vi "_Test_MMAPI_Receive.vi"() -> ()   [LabVIEW 2023]
uses:
  Shared/SensorInfos.ctl
  Shared/SensorInfo.ctl
  Shared/Sensor Name.ctl
  Shared/Protocol.ctl
  MM/MM Data.ctl
  MM/MM Objects.ctl
  MM/MM Object.ctl
  <vilib>/Utility/xml.llb/Read From XML File(string).vi
  <vilib>/xnet/xnet.llb/XNET Convert (Frame FlexRay to Signal).vi
  RDB/RDB.lvlib
  Shared/Vires VTD Shared.lvlib
  MM/MM.lvlib
  Utility/Debug_Logger/LoggingProber.lvlib
panel:
  in  "mmanager":path=path "C:/dev/Hexagon-VTD-Custom-Device/Libraries/libMM.dll"
  out "sensorInfos":T1
  out "size(s) 2":i32
  out "Array 2":u8[](array[numeric])
  out "Array":i32[](array[numeric])
  out "signal data":dbl[](array[numeric])
  out "simTime":dbl
  out "simFrame":dbl
  in  "XML File Path":path=path "C:/Debug/MM.xml"
  out "error out":errorcluster
  in  "error in (no error)":errorcluster
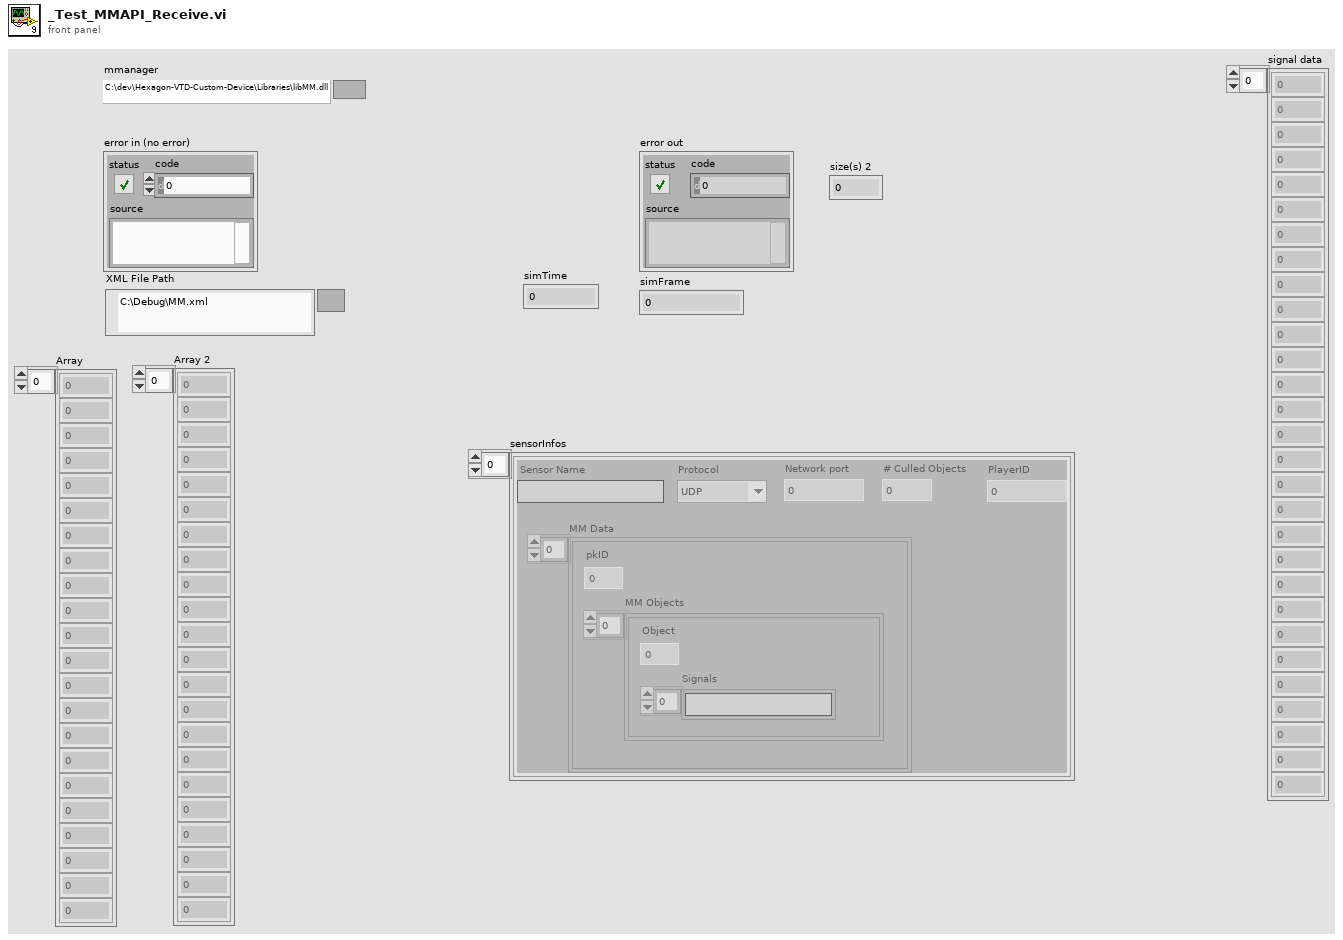
[diagram p1: front panel]
types:
  T1 = typedef "Vires VTD Shared.lvlib/SensorInfos.ctl" = T2[]
  T2 = typedef "Vires VTD Shared.lvlib/SensorInfo.ctl" = cluster{"Sensor Name":T3, "Protocol":T4, "Network port":i32, "# Culled Objects":i32, "PlayerID":u8, "MM Data":T5}
  T3 = typedef "Vires VTD Shared.lvlib/Sensor Name.ctl" = string
  T4 = typedef "Vires VTD Shared.lvlib/Protocol.ctl" = enum16{"UDP", "TCP"}
  T5 = typedef "Vires VTD Shared.lvlib/MM Data.ctl" = T6[]
  T6 = typedef "MM.lvlib/MM Objects.ctl" = cluster{"pkID":i32, "MM Objects":T7[]}
  T7 = typedef "MM.lvlib/MM Object.ctl" = cluster{"Object":i32, "Signals":string[]}
  T8 = typedef "MM.lvlib/Sensor Engine Data.ctl" = cluster{"TCP Network":refnum<k5>, "UDP Network":refnum<k16>, "Network port":i32, "Protocol":T4, "Sensor Name":T3, "Signal Data":dbl[], "MM Frames":T9[], "MM Culled Objects":i32[], "MM Frame Refs":refnum<k21>[], "mmanager":path, "mmHandle":u64}
  T9 = typedef "XNET Frame FlexRay.ctl" = cluster{"timestamp":timestamp, "payload":u8[], "slot":u16, "type":T10, "cycle count":u8, "startup?":bool, "sync?":bool, "preamble?":bool, "ch A":bool, "ch B":bool, "echo?":bool}
  T10 = typedef "XNET Frame Type FlexRay.ctl" = u8
  T11 = enum16{"Standard", "Buffered", "CRLF", "Immediate"}
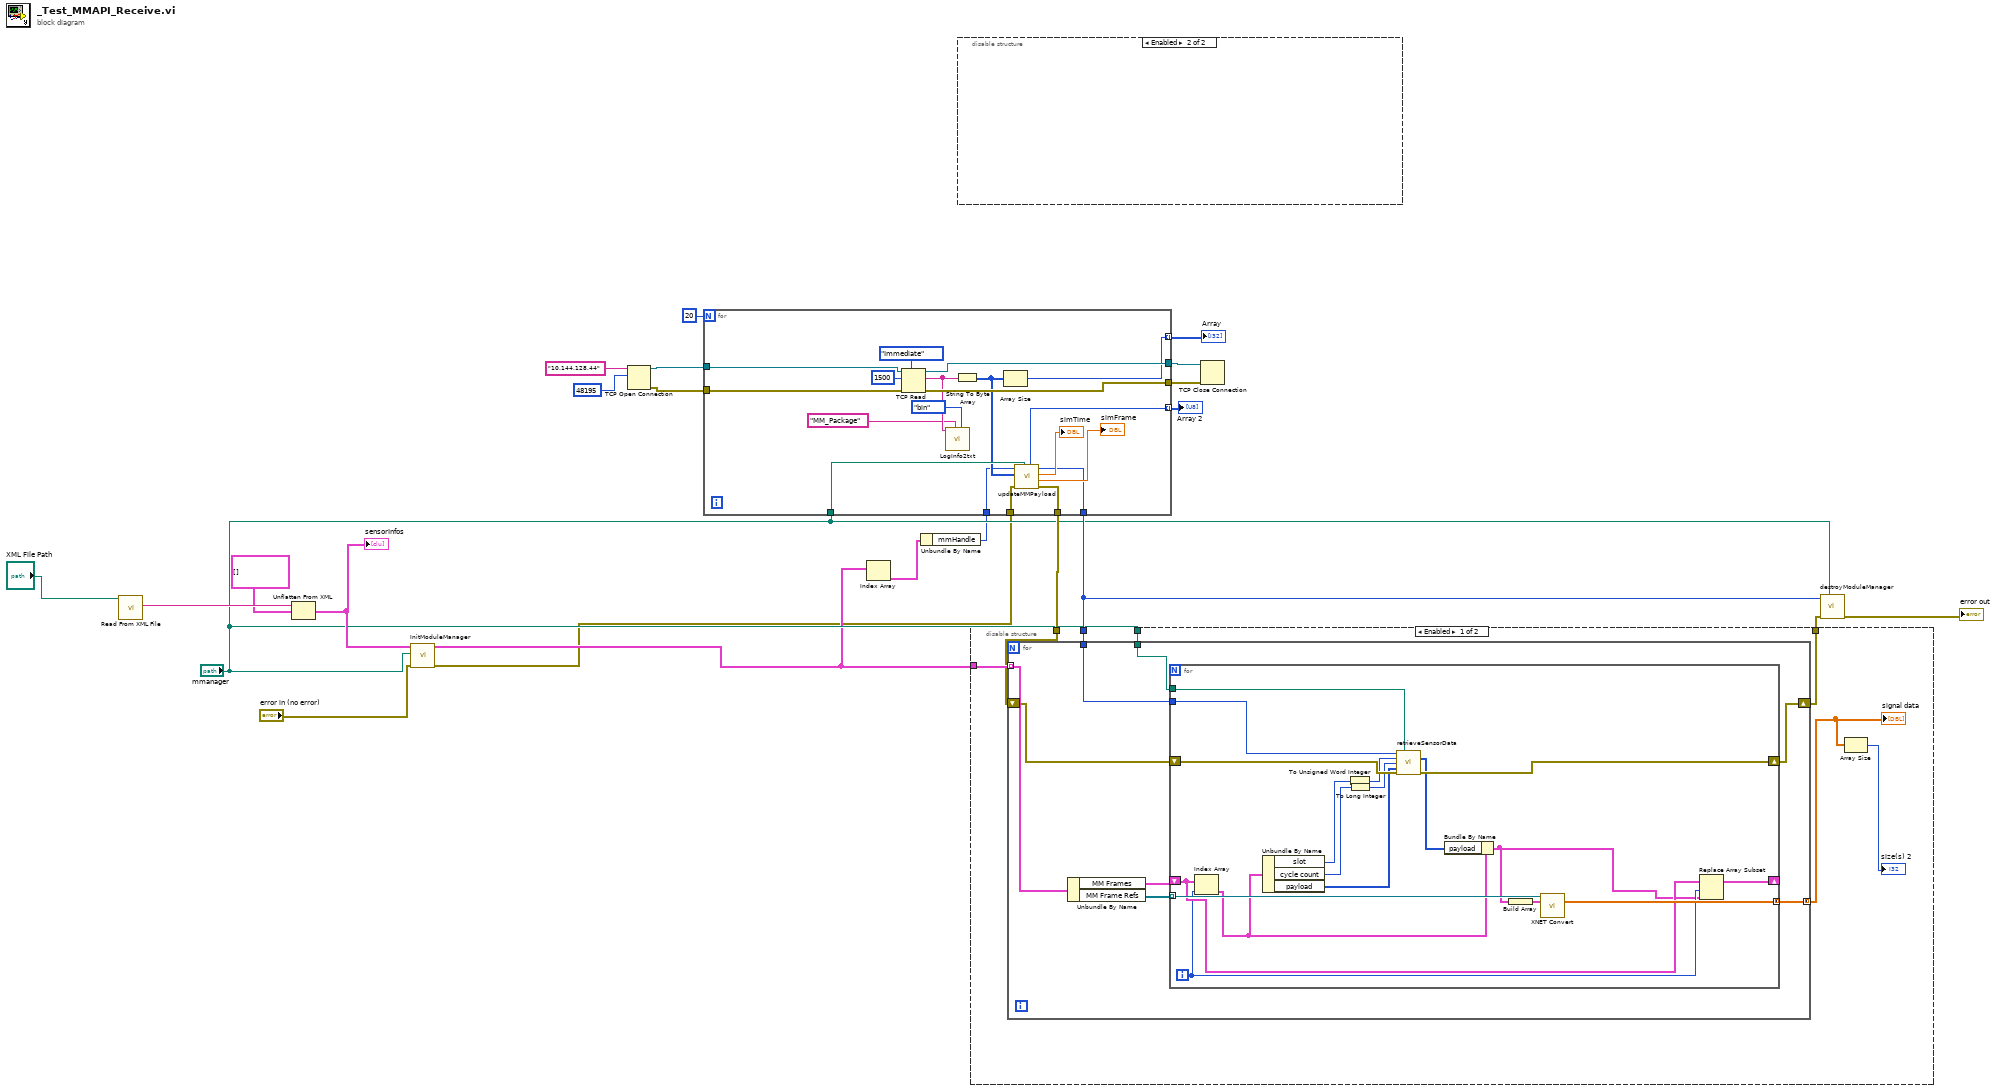
[diagram p0: block diagram]
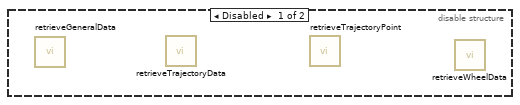
[diagram p3: hidden frame]
diagram:
  n1 = call-poly <vilib>:"Read From XML File.vi"("XML File Path"="XML File Path") -> ("XML Elements"=w23:string)  [unwired: 8 in, 2 out]
  n2 = Unflatten From XML(xml string=w23, type=T1 [] ("SensorInfos")) -> (value=w12:T1)  [unwired: 1 in, 1 out]
  "sensorInfos" <- w12
  n3 = call "InitModuleManager.vi"("error in (no error)"="error in (no error)", "mmanager"="mmanager", "SensorInfos"=w12) -> ("error out (no error)"=w1:errorcluster, "Sensor Engine Datas"=w5:T8[])  [unwired: 7 in]
  n4 = TCP Open Connection(address="10.144.128.44", remote port or service name=u16 48195) -> (connection ID=w18:refnum<k5>, error out=w19:errorcluster)  [unwired: 3 in]
  n5 = Index Array(array=w5) -> (element=w4:T8)  [unwired: 1 in]
  n6 = Unbundle By Name(w4) -> ("mmHandle"=w3:u64)
  n7 = for {
    N: 20 -> [_]
    tunnel: "mmanager" -> [w35]
    tunnel: w19 -> [w40]
    tunnel: w18 -> [w39]
    tunnel: [w38] -> w17
    tunnel: [w37] -> w16
    tunnel: [w36] -> w14 mode=indexing
    tunnel: w1 -> [w34]
    tunnel: [w32] -> w11 mode=indexing
    tunnel: [w29] -> w10
    tunnel: [w28] -> w7
    tunnel: w3 -> [w27]
    n8 = TCP Read(connection ID=w39, bytes to read=1500, error in (no error)=w40, 7:T11."Immediate" ("mode (standard)")) -> (connection ID out=w38:refnum<k5>, data out=w26:string, error out=w37:errorcluster)  [unwired: 1 in]
    n9 = call "LogInfo2txt.vi"("type"=enum16{"txt", "bin"}."bin", "File ID"="MM_Package", "text"=w26) -> ()  [unwired: 9 in]
    n10 = String To Byte Array(string=w26) -> (unsigned byte array=w33:u8[])
    n11 = Array Size(array=w33) -> (size(s)=w36:i32)
    n12 = call "updateMMPayload.vi"("path in"=w35, "error in (no error)"=w34, "payload"=w33, "mmHandle in"=w27) -> ("error out"=w29:errorcluster, "simFrame"=→"simFrame":dbl, "simTime"=→"simTime":dbl, "mmHandle out"=w28:u64, "isComplete"=w32:u8)  [unwired: 2 in, 1 out]
  }
  "Array" <- w14
  "Array 2" <- w11
  n13 = disable-structure shown="Enabled" {
    frame Disabled {
      n14 = call "retrieveGeneralData.vi"() -> ()  [unwired: 13 in, 3 out]
      n15 = call "retrieveTrajectoryData.vi"() -> ()  [unwired: 13 in, 3 out]
      n16 = call "retrieveTrajectoryPoint.vi"() -> ()  [unwired: 13 in, 3 out]
      n17 = call "retrieveWheelData.vi"() -> ()  [unwired: 13 in, 3 out]
    }
    frame Enabled {
    }
  }
  n18 = disable-structure shown="Enabled" {
    disable-tunnel: "mmanager" -> [w49 _]
    disable-tunnel: w10 -> [w46 w76]
    disable-tunnel: [w44 w76] -> w9
    disable-tunnel: w5 -> [w47 _]
    disable-tunnel: w7 -> [w45 _]
    frame Enabled {
      n19 = for {
        shift-right: [w51] -> w44
        shift-left: w46 -> [w54]
        tunnel: w49 -> [w53]
        tunnel: w47 -> [w57] mode=indexing
        tunnel: w45 -> [w52]
        tunnel: [w50] -> w43 mode=concatenating
        n20 = Unbundle By Name(w57) -> ("MM Frames"=w55:T9[], "MM Frame Refs"=w56:refnum<k21>[])
        n21 = for {
          tunnel: [w73] -> w50 mode=concatenating
          shift-right: [w74] -> w51
          shift-left: w54 -> [w75]
          tunnel: w56 -> [w72] mode=indexing
          shift-right: [w70] -> _
          shift-left: w55 -> [w69]
          tunnel: w53 -> [w66]
          tunnel: w52 -> [w65]
          i -> [w68]
          n22 = Index Array(array=w69, index=w68) -> (element=w71:T9)
          n23 = Unbundle By Name(w71) -> ("slot"=w63:u16, "cycle count"=w62:u8, "payload"=w59:u8[])
          n24 = To Unsigned Word Integer(number=w63) -> (unsigned 16bit integer=w61:u16)
          n25 = To Long Integer(number=w62) -> (32bit integer=w60:i32)
          n26 = call "retrieveSensorData.vi"("mmHandle in"=w65, "path in"=w66, "packageID"=w61, "objIndex"=w60, "dataOut"=w59, "error in (no error)"=w75) -> ("dataOut"=w58:u8[], "error out"=w74:errorcluster)  [unwired: 7 in, 1 out]
          n27 = Bundle By Name(cluster=w71, "payload"=w58) -> (w67:T9)
          n28 = Build Array(w67) -> (w64:T9[])
          n29 = call-poly <vilib>:"XNET Convert.vi"("session in"=w72, "frame data"=w64) -> ("signal data"=w73:dbl[])  [unwired: 11 in, 2 out]
          n30 = Replace Array Subset(array=w69, new element=w67, index=w68) -> (w70:T9[])
        }
      }
      "signal data" <- w43
      n31 = Array Size(array=w43) -> (size(s)=→"size(s) 2":i32)
    }
    frame Disabled {
    }
  }
  n32 = TCP Close Connection(connection ID=w17, error in (no error)=w16) -> ()  [unwired: 1 in, 2 out]
  n33 = call "destroyModuleManager.vi"("path in"="mmanager", "error in (no error)"=w9, "mmHandle"=w7) -> ("error out"=→"error out":errorcluster)  [unwired: 8 in]
